vi "create setpoint list.vi"(11 "error in (no error)":errorcluster) -> (1 "N points":i32=5, 6 "Setpoint array":dbl[](array[numeric])=[40.0, 50.0, 60.0, 50.0, 40.0], 15 "error out":errorcluster)   [LabVIEW 2019]
doc: "This is a Bug C(T) subVI.\n\nThis popup subvi lets the user of the bug experiment create a list of setpoints for the experiment.\n\nPaul K Dixon\nP3600\nCSUSB Physics"
uses:
  globals/Bug globals.vi
panel:
  in  "N intervals hold":i32=2
  out "Experimental Temperature Profile":dbl[](graph)=[40.0, 50.0, 60.0, 50.0, 40.0]
  in  "stop":bool
  in  "N intervals ramp":i32=2
  in  "end temp (C)":dbl=60.0
  in  "start temp (C)":dbl=40.0
  # "Create Setpoint List"
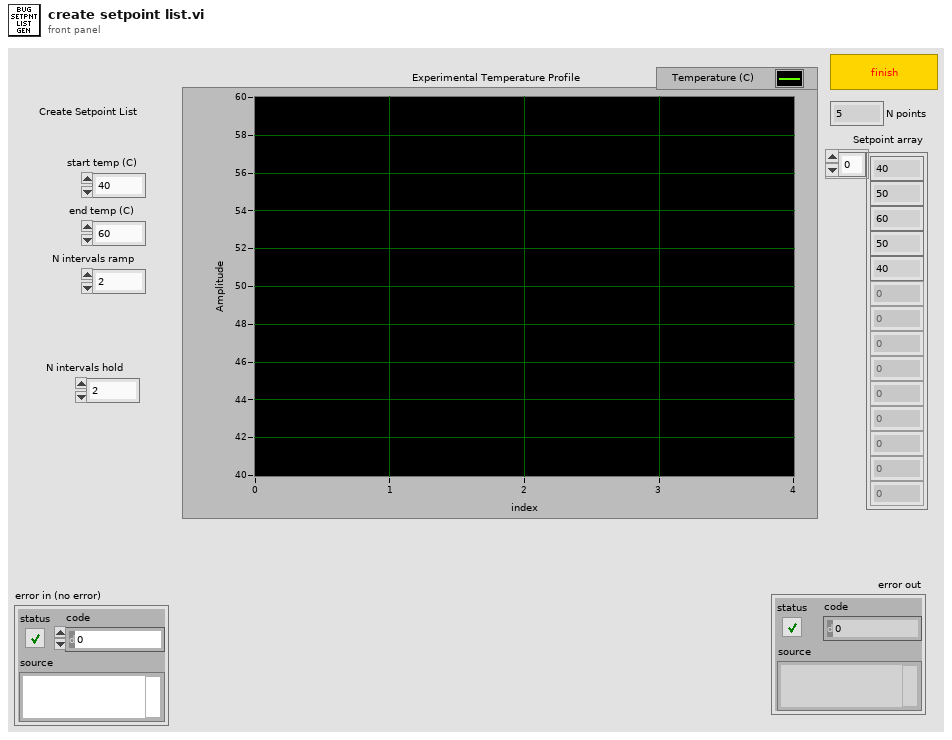
[diagram p1: front panel]
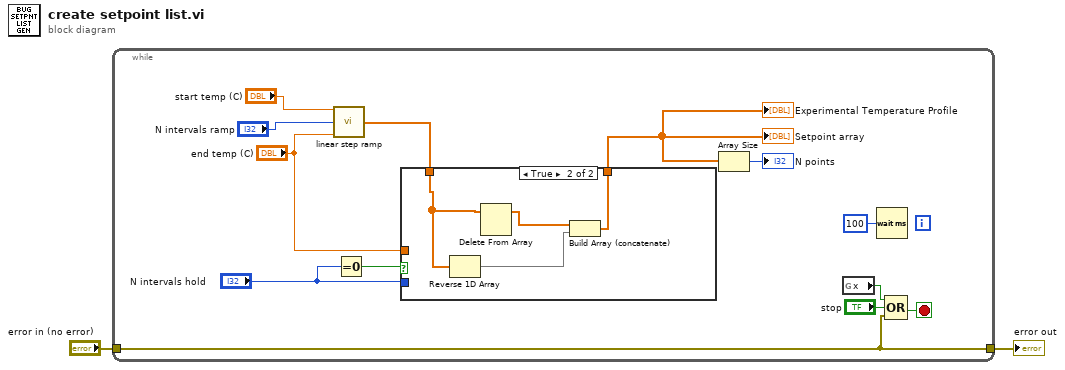
[diagram p0: block diagram]
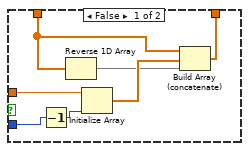
[diagram p2: hidden frame]
diagram:
  n1 = while {
    tunnel: "error in (no error)" -> [w12]
    tunnel: [w12] -> w1
    stop <- w13 stop-if-true
    n2 = call "linear step ramp.vi"("start"="start temp (C)", "N ramps"="N intervals ramp", "End"="end temp (C)") -> ("Vakues array"=w7:dbl[])  [unwired: 10 in, 2 out]
    n3 = Equal To 0?(x="N intervals hold") -> (x = 0?=w3:bool)
    n4 = case shown="True" w3 {
      tunnel: [w16 w26] -> w6
      tunnel: w7 -> [w19 w25]
      tunnel: "N intervals hold" -> [w22 _]
      tunnel: "end temp (C)" -> [w20 _]
      frame False {
        n5 = Decrement(x=w22) -> (x-1=w21:i32)
        n6 = Reverse 1D Array(array=w19) -> (reversed array=w17:dbl[])
        n7 = Initialize Array(w20, w21) -> (w18:dbl[])
        n8 = Build Array (concatenate)(w19, w18, w17) -> (w16:dbl[])
      }
      frame True {
        n9 = Reverse 1D Array(array=w25) -> (reversed array=w24:dbl[])
        n10 = Delete From Array(array=w25) -> (array with subset deleted=w23:dbl[])  [unwired: 2 in, 1 out]
        n11 = Build Array (concatenate)(w23, w24) -> (w26:dbl[])
      }
    }
    "Setpoint array" <- w6
    "Experimental Temperature Profile" <- w6
    n12 = Array Size(array=w6) -> (size(s)=→"N points":i32)
    n13 = global read "Bug globals.vi" "x"() -> (w10:bool)
    n14 = Wait (ms)(milliseconds to wait=u32 100) -> ()  [unwired: 1 out]
    n15 = Compound Arithmetic op=OR(w10, "stop", w12) -> (w13:bool)
  }
  "error out" <- w1
